vi "Comparer.vi"(5 "Resource name":string) -> (1 "Boolean":bool=TRUE, 2 "Resource name":string)   [LabVIEW 2011]
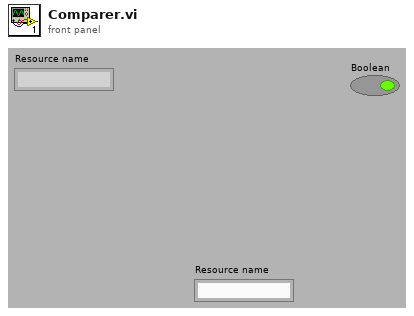
[diagram p1: front panel]
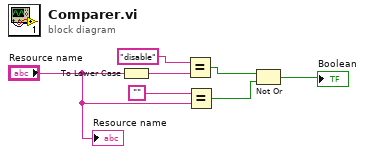
[diagram p0: block diagram]
diagram:
  n1 = To Lower Case(string="Resource name") -> (all lower case string=w6:string)
  n2 = Equal?(x="disable", y=w6) -> (x = y?=w3:bool)
  n3 = Equal?(x="", y="Resource name") -> (x = y?=w4:bool)
  n4 = Not Or(1:w4, 2:w3) -> (0:→"Boolean":bool)
  "Resource name" <- "Resource name"
